vi "Periodic Tasks.vi"() -> ()   [LabVIEW 2012]
doc: "This VI runs in parallel to other tasks. It can contain as many user-defined periodic loops as you need. These can carry out PID or other sorts of timed response."
uses:
  <vilib>/Rock Robotics/SystemInterfaces/Utilities/FPGA_UtilitiesLED Source.ctl
  <vilib>/Rock Robotics/SystemInterfaces/Utilities/FPGA_UtilitiesLED State.ctl
  Robot Global Data.vi
panel:
  in  "Use DS Data":bool
  in  "Reset REncoder":bool
  in  "Reset LEncoder":bool
  out "RDist":dbl
  out "RDir":bool
  out "RRate":dbl
  in  "Shoot Deadband":dbl=0.05
  out "Angular Rate":dbl
  out "Angle":dbl
  out "LRate":dbl
  out "LDir":bool
  out "LDist":dbl
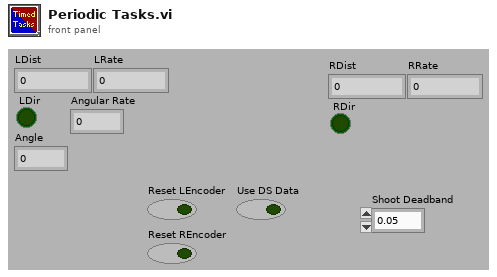
[diagram p1: front panel]
types:
  T1 = typedef "FPGA_UtilitiesLED State.ctl" = enum16{"Off", "On", "Toggle"}
  T2 = typedef "FPGA_UtilitiesLED Source.ctl" = enum16{"User LED", "FPGA LED"}
  T3 = cluster{"ClimbManualExt":dbl, "ClimbManualDep":dbl, "ClimbRetEnable":bool, "ClimbPOTDep":dbl, "ClimbConst":cluster{"ClimbConstDep":dbl, "ClimbConstFold":dbl, "ClimbConstExt":dbl, "ClimbConstRet":dbl}, "ClimbPOTExt":dbl, "ClimbExtEnable":bool, "ClimbLimit":bool, "ClimbFoldEnable":bool, "ClimbDepEnable":bool, "ClimbCase":dbl}
  T4 = cluster{"ShootTrackEnable":bool, "ShootStartWheels":bool, "ShootIndexerEnable":bool, "ShootCase":dbl, "ShootPOTElev":dbl, "ShootManualElev":dbl, "IndexerSpeed":dbl, "Wheel Spd F":dbl, "Deadband":dbl, "ShootConstElev":cluster{"1":dbl, "2":dbl, "3":dbl, "4":dbl, "Ground":dbl}, "ShootRollerSpd":dbl, "ShootFlipperPE":bool, "Wheel Spd B":dbl, "ShootConstFlipper":cluster{"Down 1":dbl, "Up 1":dbl, "Up 2":dbl, "Down 2":dbl}, "Y Coord":dbl}
  T5 = typedef "WPI_DigitalInputDevRef.ctl" = cluster{"DevStatus":errorcluster, "DIO Channel":T6, "Digital Module":T7}
  T6 = typedef "FPGA_DIOChannel.ctl" = enum8{"DIO 1", "DIO 2", "DIO 3", "DIO 4", "DIO 5", "DIO 6", "DIO 7", "DIO 8", "DIO 9", "DIO 10", "DIO 11", "DIO 12", "DIO 13", "DIO 14", "Invalid"}
  T7 = typedef "FPGA_TypedefDigitalModule.ctl" = enum16{"Digital Module 1", "Digital Module 2"}
  T8 = typedef "WPI_AnalogChannelDevRef.ctl" = cluster{"DevStatus":errorcluster, "Analog Module":T9, "Analog Channel":T10}
  T9 = typedef "FPGA_TypedefAnalogModule.ctl" = enum16{"Analog Module 1", "Analog Module 2"}
  T10 = typedef "FPGA_AIChannel.ctl" = enum8{"AI 1", "AI 2", "AI 3", "AI 4", "AI 5", "AI 6", "AI 7", "AI 8", "Invalid"}
  T11 = cluster{"Down 1":dbl, "Up 1":dbl, "Up 2":dbl, "Down 2":dbl}
  T12 = cluster{"Ground":dbl, "1":dbl, "2":dbl, "3":dbl, "4":dbl}
  T13 = typedef "WPI_RelayValue.ctl" = enum16{"Off", "On", "Forward", "Reverse"}
  T14 = cluster{"Indexer":dbl, "ShooterElev":dbl, "Case":dbl, "ShooterWheelF":dbl, "ShooterWheelB":dbl, "Rollers":dbl, "Flipper":dbl, "Flipper2":dbl, "Harvestor":T13}
  T15 = typedef "WPI_GyroDevRef.ctl" = cluster{"DevStatus":errorcluster, "Analog Module":T9, "Analog Channel":T10, "Offset":dbl, "Gain (VoltsPerDegree/Second)":dbl}
  T16 = typedef "WPI_EncoderDevRef.ctl" = cluster{"DevStatus":errorcluster, "EncoderIndex":T17, "CounterIndex":T18, "DistancePerCount":dbl, "Decoding Type":T19}
  T17 = typedef "FPGA_EncoderIdx.ctl" = enum8{"Enc 0", "Enc 1", "Enc 2", "Enc 3", "Invalid"}
  T18 = typedef "FPGA_CounterCtrSystemIndex.ctl" = enum8{"Ctr 0", "Ctr 1", "Ctr 2", "Ctr 3", "Ctr 4", "Ctr 5", "Ctr 6", "Ctr 7", "Invalid"}
  T19 = typedef "WPI_EncoderType.ctl" = enum16{"1x", "2x", "4x"}
  T20 = cluster{"ClimbConstDep":dbl, "ClimbConstFold":dbl, "ClimbConstExt":dbl, "ClimbConstRet":dbl}
  T21 = cluster{"ClimbOutDep":dbl, "ClimbOutExt":dbl, "ClimbOutCase":i32}
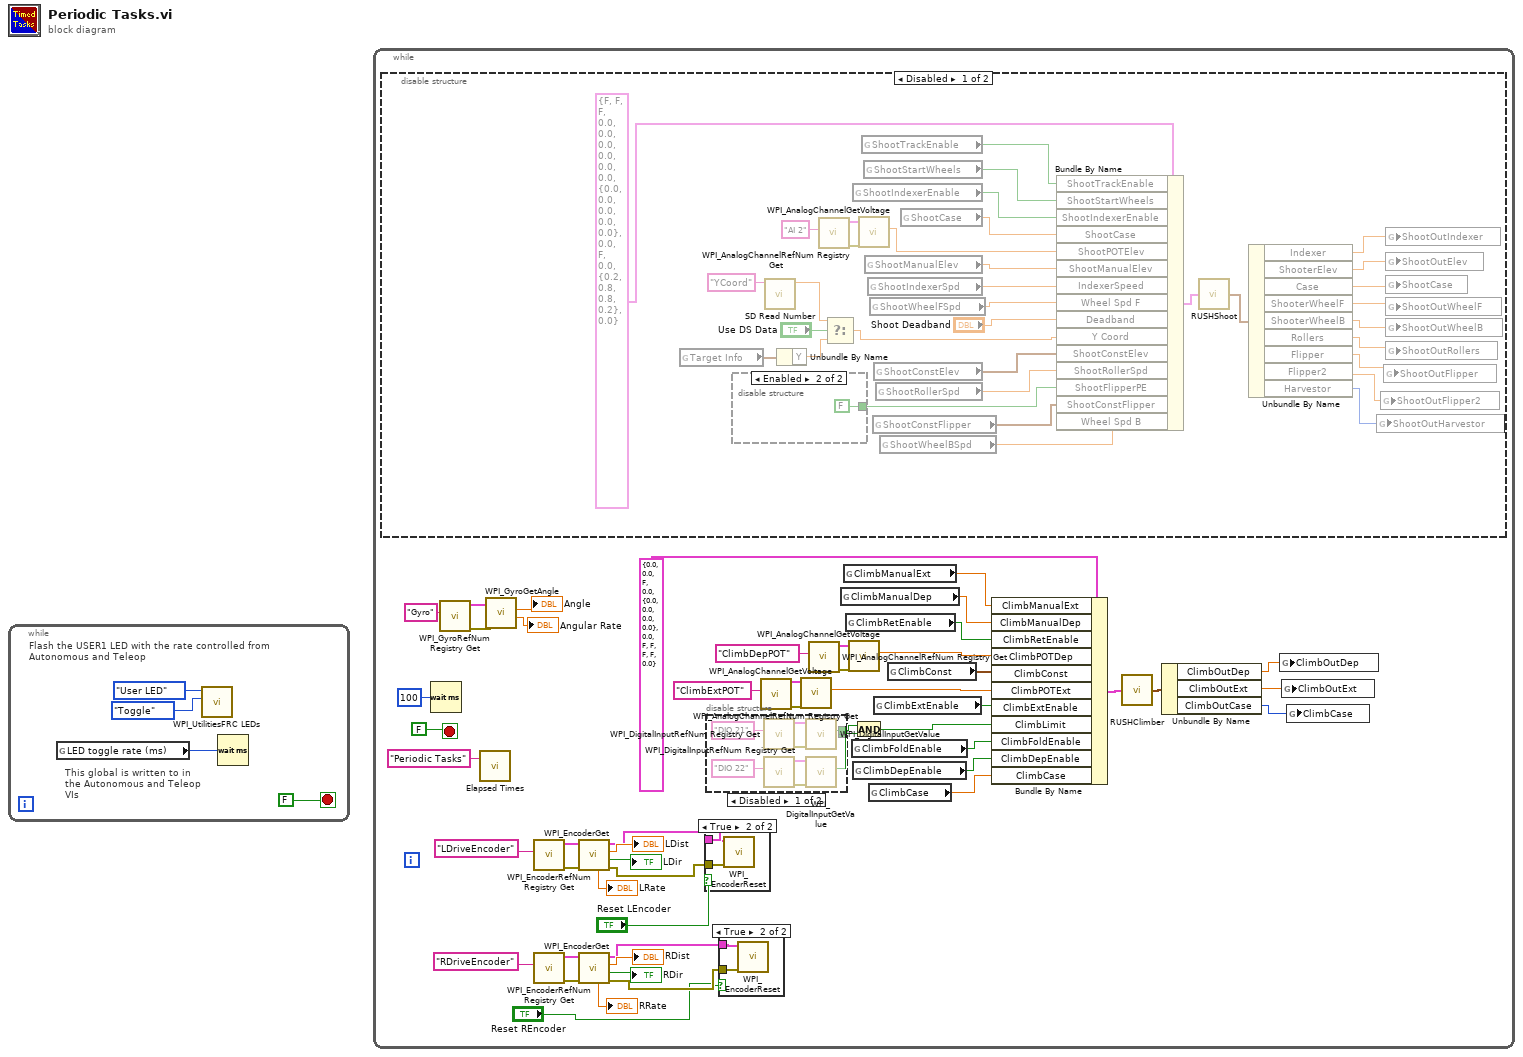
[diagram p0: block diagram]
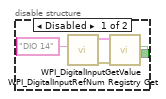
[diagram p5: hidden frame]
diagram:
  n1 = while {
    stop <- FALSE stop-if-true
    # "This global is written to in the Autonomous and Teleop VIs"
    # "Flash the USER1 LED with the rate controlled from Autonomous and Teleop"
    n2 = global read "Robot Global Data.vi" "LED toggle rate (ms)"() -> (w1:u32)
    n3 = call <vilib>:"WPI_UtilitiesFRC LEDs.vi"("State"=FPGA_UtilitiesLED_State."Toggle", "LED Type"=FPGA_UtilitiesLED_Source."User LED") -> ()  [unwired: 1 in, 9 out]
    n4 = Wait (ms)(milliseconds to wait=w1) -> ()  [unwired: 1 out]
  }
  n5 = while {
    stop <- FALSE stop-if-true
    n6 = disable-structure shown="Disabled" {
      frame Disabled {
        n7 = global read "Robot Global Data.vi" "Target Info"() -> (w73:cluster{"X":dbl, "Y":dbl, "Distance (ft)":dbl})
        n8 = disable-structure shown="Enabled" {
          disable-tunnel: [w103 FALSE ("Value")] -> w84
          frame Disabled {
            n9 = call <vilib>:"WPI_DigitalInputRefNum Registry Get.vi"("refnum name"="DIO 14") -> ("error out"=w106:errorcluster, "DigitalInputDevRef"=w105:T5)  [unwired: 9 in]
            n10 = call <vilib>:"WPI_DigitalInputGetValue.vi"("error in (no error)"=w106, "DigitalInputDevRef"=w105) -> ("Value"=w103:bool)  [unwired: 7 in, 2 out]
          }
          frame Enabled {
          }
        }
        n11 = call <vilib>:"SD Read Number.vi"("Name"="YCoord") -> ("Numeric"=w70:dbl)  [unwired: 8 in, 2 out]
        n12 = Unbundle By Name(w73) -> ("Y"=w72:dbl)
        n13 = call <vilib>:"WPI_AnalogChannelRefNum Registry Get.vi"("refnum name"="AI 2") -> ("error out"=w87:errorcluster, "AIDeviceRef"=w86:T8)  [unwired: 9 in]
        n14 = Select(t=w70, s="Use DS Data", f=w72) -> (s? t:f=w71:dbl)
        n15 = global read "Robot Global Data.vi" "ShootIndexerEnable"() -> (w96:bool)
        n16 = call <vilib>:"WPI_AnalogChannelGetVoltage.vi"("error in (no error)"=w87, "AIDeviceRef"=w86) -> ("Voltage"=w85:dbl)  [unwired: 7 in, 2 out]
        n17 = global read "Robot Global Data.vi" "ShootTrackEnable"() -> (w98:bool)
        n18 = global read "Robot Global Data.vi" "ShootStartWheels"() -> (w97:bool)
        n19 = global read "Robot Global Data.vi" "ShootManualElev"() -> (w95:dbl)
        n20 = global read "Robot Global Data.vi" "ShootIndexerSpd"() -> (w101:dbl)
        n21 = global read "Robot Global Data.vi" "ShootWheelFSpd"() -> (w100:dbl)
        n22 = global read "Robot Global Data.vi" "ShootConstFlipper"() -> (w81:T11)
        n23 = global read "Robot Global Data.vi" "ShootConstElev"() -> (w99:T12)
        n24 = global read "Robot Global Data.vi" "ShootRollerSpd"() -> (w94:dbl)
        n25 = global read "Robot Global Data.vi" "ShootWheelBSpd"() -> (w82:dbl)
        n26 = global read "Robot Global Data.vi" "ShootCase"() -> (w102:dbl)
        n27 = Bundle By Name(cluster=T4 {"ShootTrackEnable"=FALSE, "ShootStartWheels"=FALSE, "ShootIndexerEnable"=FALSE, "ShootCase"=0.0, "ShootPOTElev"=0.0, "ShootManualElev"=0.0, "IndexerSpeed"=0.0, "Wheel Spd F"=0.0, "Deadband"=0.0, "ShootConstElev"={"1"=0.0, "2"=0.0, "3"=0.0, "4"=0.0, "Ground"=0.0}, "ShootRollerSpd"=0.0, "ShootFlipperPE"=FALSE, "Wheel Spd B"=0.0, "ShootConstFlipper"={"Down 1"=0.2, "Up 1"=0.8, "Up 2"=0.8, "Down 2"=0.2}, "Y Coord"=0.0} ("In Cluster"), "ShootTrackEnable"=w98, "ShootStartWheels"=w97, "ShootIndexerEnable"=w96, "ShootCase"=w102, "ShootPOTElev"=w85, "ShootManualElev"=w95, "IndexerSpeed"=w101, "Wheel Spd F"=w100, "Deadband"="Shoot Deadband", "Y Coord"=w71, "ShootConstElev"=w99, "ShootRollerSpd"=w94, "ShootFlipperPE"=w84, "ShootConstFlipper"=w81, "Wheel Spd B"=w82) -> (w68:T4)
        n28 = call "RUSHShoot.vi"("In Cluster"=w68) -> ("Out Cluster"=w93:T14)
        n29 = Unbundle By Name(w93) -> ("Indexer"=w90:dbl, "ShooterElev"=w91:dbl, "Case"=w92:dbl, "ShooterWheelF"=w89:dbl, "ShooterWheelB"=w80:dbl, "Rollers"=w79:dbl, "Flipper"=w78:dbl, "Flipper2"=w77:dbl, "Harvestor"=w76:T13)
        n30 = global write "Robot Global Data.vi" "ShootOutHarvestor"(w76) -> ()
        n31 = global write "Robot Global Data.vi" "ShootOutFlipper2"(w77) -> ()
        n32 = global write "Robot Global Data.vi" "ShootOutFlipper"(w78) -> ()
        n33 = global write "Robot Global Data.vi" "ShootOutIndexer"(w90) -> ()
        n34 = global write "Robot Global Data.vi" "ShootOutElev"(w91) -> ()
        n35 = global write "Robot Global Data.vi" "ShootCase"(w92) -> ()
        n36 = global write "Robot Global Data.vi" "ShootOutWheelF"(w89) -> ()
        n37 = global write "Robot Global Data.vi" "ShootOutWheelB"(w80) -> ()
        n38 = global write "Robot Global Data.vi" "ShootOutRollers"(w79) -> ()
      }
      frame Enabled {
      }
    }
    n39 = Wait (ms)(milliseconds to wait=u32 100) -> ()  [unwired: 1 out]
    n40 = call <vilib>:"WPI_GyroRefNum Registry Get.vi"("refnum name"="Gyro") -> ("error out"=w48:errorcluster, "GyroDevRef"=w49:T15)  [unwired: 9 in]
    n41 = call "Elapsed Times.vi"("Call Name"="Periodic Tasks") -> ()  [unwired: 2 in, 1 out]
    n42 = call <vilib>:"WPI_GyroGetAngle.vi"("error in (no error)"=w48, "GyroDevRef"=w49) -> ("Angular Rate"=→"Angular Rate":dbl, "Angle"=→"Angle":dbl)  [unwired: 6 in, 2 out]
    n43 = call <vilib>:"WPI_EncoderRefNum Registry Get.vi"("refnum name"="LDriveEncoder") -> ("error out"=w20:errorcluster, "EncoderDevRef"=w21:T16)  [unwired: 9 in]
    n44 = call <vilib>:"WPI_EncoderRefNum Registry Get.vi"("refnum name"="RDriveEncoder") -> ("error out"=w19:errorcluster, "EncoderDevRef"=w18:T16)  [unwired: 9 in]
    n45 = call <vilib>:"WPI_EncoderGet.vi"("error in (no error)"=w20, "EncoderDevRef"=w21) -> ("error out"=w12:errorcluster, "Direction"=→"LDir":bool, "Distance"=→"LDist":dbl, "EncoderDevRef"=w13:T16, "Rate"=→"LRate":dbl)  [unwired: 4 in, 1 out]
    n46 = call <vilib>:"WPI_EncoderGet.vi"("error in (no error)"=w19, "EncoderDevRef"=w18) -> ("error out"=w10:errorcluster, "Direction"=→"RDir":bool, "Distance"=→"RDist":dbl, "EncoderDevRef"=w9:T16, "Rate"=→"RRate":dbl)  [unwired: 4 in, 1 out]
    n47 = case shown="True" "Reset LEncoder" {
      tunnel: w13 -> [_ w59]
      tunnel: w12 -> [_ w58]
      frame False {
      }
      frame True {
        n48 = call <vilib>:"WPI_EncoderReset.vi"("error in (no error)"=w58, "EncoderDevRef"=w59) -> ()  [unwired: 8 in, 2 out]
      }
    }
    n49 = disable-structure shown="Disabled" {
      disable-tunnel: [w67 _] -> w44
      disable-tunnel: [w66 _] -> w43
      frame Disabled {
        n50 = call <vilib>:"WPI_DigitalInputRefNum Registry Get.vi"("refnum name"="DIO 21") -> ("error out"=w63:errorcluster, "DigitalInputDevRef"=w64:T5)  [unwired: 9 in]
        n51 = call <vilib>:"WPI_DigitalInputRefNum Registry Get.vi"("refnum name"="DIO 22") -> ("error out"=w62:errorcluster, "DigitalInputDevRef"=w61:T5)  [unwired: 9 in]
        n52 = call <vilib>:"WPI_DigitalInputGetValue.vi"("error in (no error)"=w63, "DigitalInputDevRef"=w64) -> ("Value"=w66:bool)  [unwired: 7 in, 2 out]
        n53 = call <vilib>:"WPI_DigitalInputGetValue.vi"("error in (no error)"=w62, "DigitalInputDevRef"=w61) -> ("Value"=w67:bool)  [unwired: 7 in, 2 out]
      }
      frame Enabled {
      }
    }
    n54 = case shown="True" "Reset REncoder" {
      tunnel: w9 -> [_ w57]
      tunnel: w10 -> [_ w56]
      frame False {
      }
      frame True {
        n55 = call <vilib>:"WPI_EncoderReset.vi"("error in (no error)"=w56, "EncoderDevRef"=w57) -> ()  [unwired: 8 in, 2 out]
      }
    }
    n56 = call <vilib>:"WPI_AnalogChannelRefNum Registry Get.vi"("refnum name"="ClimbExtPOT") -> ("error out"=w6:errorcluster, "AIDeviceRef"=w5:T8)  [unwired: 9 in]
    n57 = call <vilib>:"WPI_AnalogChannelGetVoltage.vi"("error in (no error)"=w6, "AIDeviceRef"=w5) -> ("Voltage"=w37:dbl)  [unwired: 7 in, 2 out]
    n58 = call <vilib>:"WPI_AnalogChannelRefNum Registry Get.vi"("refnum name"="ClimbDepPOT") -> ("error out"=w41:errorcluster, "AIDeviceRef"=w39:T8)  [unwired: 9 in]
    n59 = global read "Robot Global Data.vi" "ClimbManualDep"() -> (w35:dbl)
    n60 = global read "Robot Global Data.vi" "ClimbManualExt"() -> (w36:dbl)
    n61 = global read "Robot Global Data.vi" "ClimbRetEnable"() -> (w34:bool)
    n62 = call <vilib>:"WPI_AnalogChannelGetVoltage.vi"("error in (no error)"=w41, "AIDeviceRef"=w39) -> ("Voltage"=w38:dbl)  [unwired: 7 in, 2 out]
    n63 = global read "Robot Global Data.vi" "ClimbFoldEnable"() -> (w31:bool)
    n64 = global read "Robot Global Data.vi" "ClimbDepEnable"() -> (w30:bool)
    n65 = And(x=w43, y=w44) -> (x .and. y?=w42:bool)
    n66 = global read "Robot Global Data.vi" "ClimbCase"() -> (w29:dbl)
    n67 = global read "Robot Global Data.vi" "ClimbExtEnable"() -> (w32:bool)
    n68 = global read "Robot Global Data.vi" "ClimbConst"() -> (w33:T20)
    n69 = Bundle By Name(cluster=T3 {"ClimbManualExt"=0.0, "ClimbManualDep"=0.0, "ClimbRetEnable"=FALSE, "ClimbPOTDep"=0.0, "ClimbConst"={"ClimbConstDep"=0.0, "ClimbConstFold"=0.0, "ClimbConstExt"=0.0, "ClimbConstRet"=0.0}, "ClimbPOTExt"=0.0, "ClimbExtEnable"=FALSE, "ClimbLimit"=FALSE, "ClimbFoldEnable"=FALSE, "ClimbDepEnable"=FALSE, "ClimbCase"=0.0} ("In Cluster 2"), "ClimbManualExt"=w36, "ClimbManualDep"=w35, "ClimbRetEnable"=w34, "ClimbPOTDep"=w38, "ClimbConst"=w33, "ClimbPOTExt"=w37, "ClimbExtEnable"=w32, "ClimbLimit"=w42, "ClimbFoldEnable"=w31, "ClimbDepEnable"=w30, "ClimbCase"=w29) -> (w46:T3)
    n70 = call "RUSHClimber.vi"("In Cluster"=w46) -> ("Out Cluster"=w45:T21)
    n71 = Unbundle By Name(w45) -> ("ClimbOutDep"=w26:dbl, "ClimbOutExt"=w27:dbl, "ClimbOutCase"=w28:i32)
    n72 = global write "Robot Global Data.vi" "ClimbOutDep"(w26) -> ()
    n73 = global write "Robot Global Data.vi" "ClimbOutExt"(w27) -> ()
    n74 = global write "Robot Global Data.vi" "ClimbCase"(w28) -> ()
  }
